vi "旋转臂角度读取-子.vi"(0 "error out":errorcluster caption="错误输出", 2 "task out 2":refnum<k21> caption="任务输出") -> (1 "旋转臂角度":dbl)   [LabVIEW 2015]
uses:
  <vilib>/DAQmx/read.llb/DAQmx Read (Counter U32 1Chan 1Samp).vi
  <vilib>/DAQmx/miscellaneous.llb/DAQmx Fill In Error Info.vi
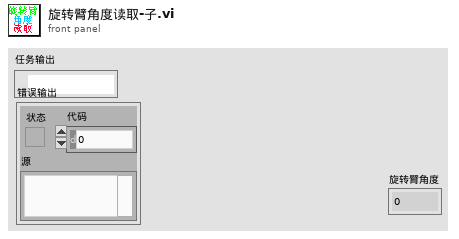
[diagram p1: front panel]
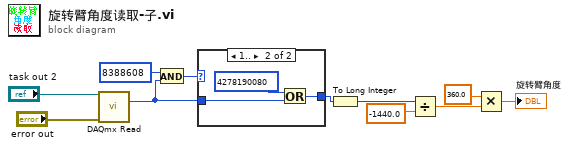
[diagram p0: block diagram]
diagram:
  n1 = call-poly <vilib>:"DAQmx Read.vi"("task/channels in"="task out 2", "error in"="error out") -> ("data"=w1:u32)  [unwired: 11 in, 2 out]
  n2 = And(x=u32 8388608, y=w1) -> (x .and. y?=w4:u32)
  n3 = case shown="1.." w4 {
    tunnel: w1 -> [w12 w15]
    tunnel: [w12 w13] -> w2
    frame ..0 {
    }
    frame 1.. {
      n4 = Or(x=u32 4278190080, y=w15) -> (x .or. y?=w13:u32)
    }
  }
  n5 = To Long Integer(number=w2) -> (32bit integer=w7:i32)
  n6 = Divide(x=w7, y=-1440.0) -> (x/y=w10:dbl)
  n7 = Multiply(x=360.0, y=w10) -> (x*y=→"旋转臂角度":dbl)
